vi "Analysis Test.vi"() -> ()   [LabVIEW 2017]
uses:
  Controller/Controller Data Cluster.ctl
  User Console/UI Data Cluster.ctl
  Controller/Timed Action.ctl
  Controller/Current Direction.ctl
  Controller/Communication/Controller Queue Message.ctl
panel:
  out "Current Direction":T1
  out "Controller Queue Message":T2=enum."Start and Move"
  in  "Controller Data Cluster 2":T3={"UI Data Cluster"={"Floor Selection"=[], "Elevator Call Up"=[], "Elevator Call Down"=[], "Door Buttons"={"Open"=FALSE, "Close"=FALSE}, "Emergency"=FALSE}, "Sensor Position"=1, "Module Closed?"={"Display Loop"=FALSE, "Sensor Loop "=FALSE}, "Time to Elapse"=0, "Request?"=FALSE, "Timed Action"=enum."Open Door", "Time Constants"={"Open Door"=5.0, "Close Door"=1.0, "Travel"=10.0, "Inactivity"=20.0}, "Inactivity"=FALSE, "Current Floor"=1, "Current Direction"=enum."Idle", "Travel?"=FALSE, "Program Exit"=[], "Emergency?"=FALSE}
  out "Error In 2":errorcluster
  in  "Error In":errorcluster
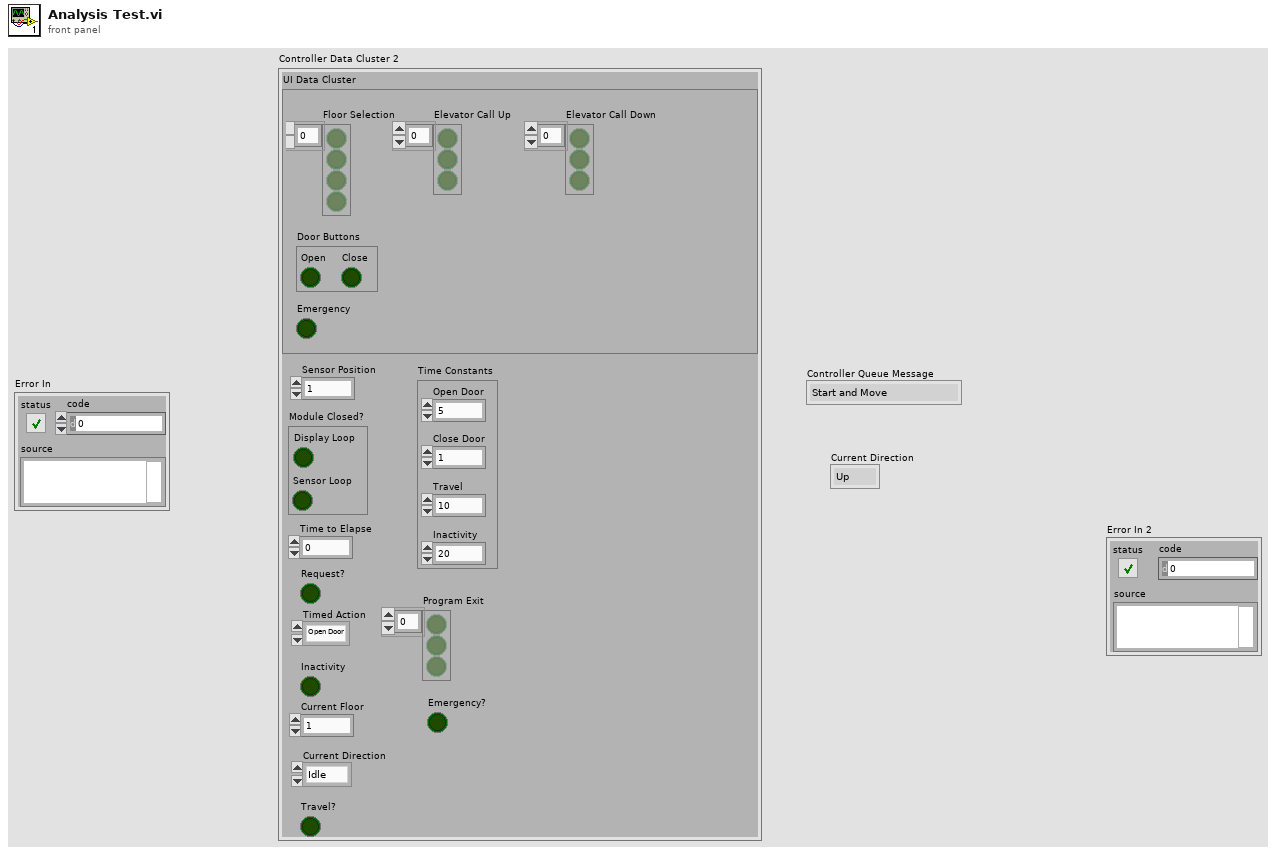
[diagram p1: front panel]
types:
  T1 = typedef "Current Direction.ctl" = enum16{"Up", "Down", "Idle"}
  T2 = typedef "Controller Queue Message.ctl" = enum16{"Initialize", "User Console Update", "Sensor Update", "Wait for First Request", "Start and Move", "Analysis", "Continue Travel", "Stop at Floor", "Open and Close Door Sequence", "Close Door", "No Request Remaining", "Check Time", "Emergency Call", "Terminate Process", "Start Exit", "Error Handling"}
  T3 = typedef "Controller Data Cluster.ctl" = cluster{"UI Data Cluster":T4, "Sensor Position":u32, "Module Closed?":cluster{"Display Loop":bool, "Sensor Loop ":bool}, "Time to Elapse":u32, "Request?":bool, "Timed Action":T5, "Time Constants":cluster{"Open Door":dbl, "Close Door":dbl, "Travel":dbl, "Inactivity":dbl}, "Inactivity":bool, "Current Floor":u32, "Current Direction":T1, "Travel?":bool, "Program Exit":bool[], "Emergency?":bool}
  T4 = typedef "UI Data Cluster.ctl" = cluster{"Floor Selection":bool[], "Elevator Call Up":bool[], "Elevator Call Down":bool[], "Door Buttons":cluster{"Open":bool, "Close":bool}, "Emergency":bool}
  T5 = typedef "Timed Action.ctl" = enum16{"Open Door", "Close Door", "Travel", "Inactivity"}
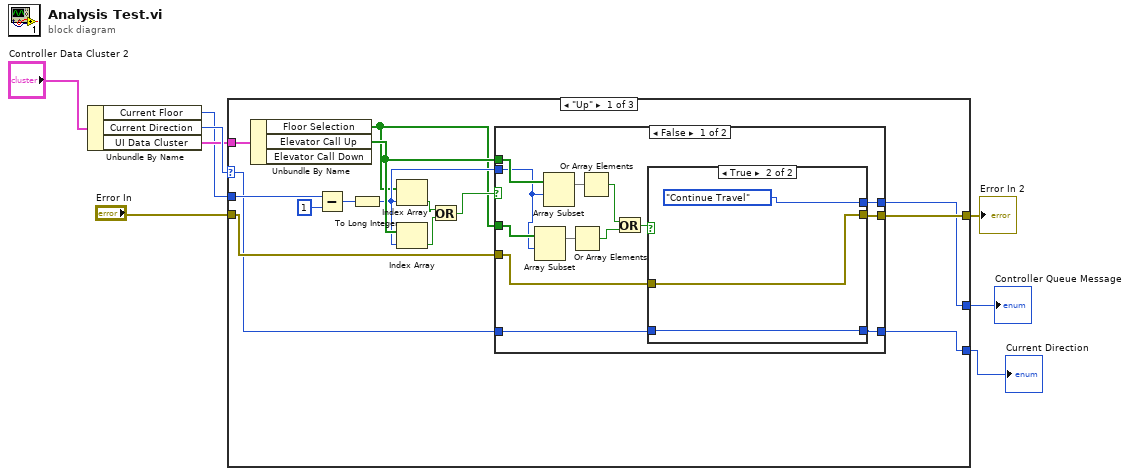
[diagram p0: block diagram]
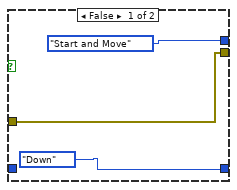
[diagram p2: hidden frame]
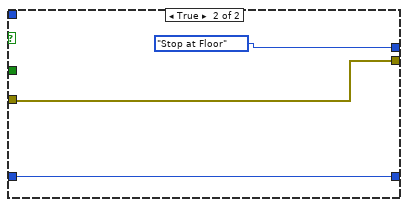
[diagram p3: hidden frame]
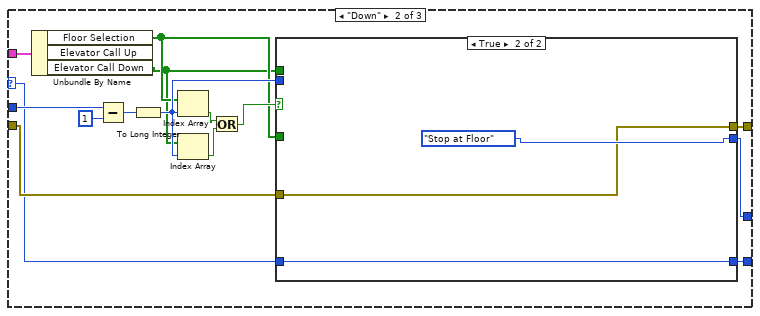
[diagram p4: hidden frame]
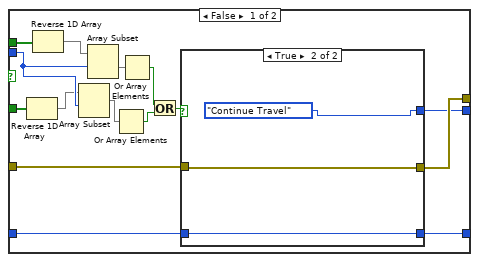
[diagram p5: hidden frame]
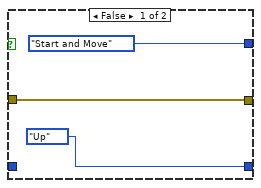
[diagram p6: hidden frame]
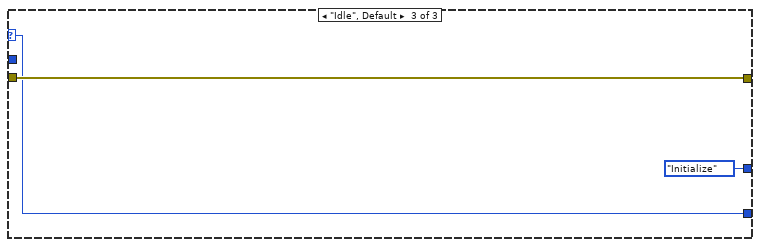
[diagram p7: hidden frame]
diagram:
  n1 = Unbundle By Name("Controller Data Cluster 2") -> ("Current Floor"=w6:u32, "Current Direction"=w8:T1, "UI Data Cluster"=w7:T4)
  n2 = case shown="\"Up\"" w8 {
    selector: w8 -> [w9 w46 w85]
    tunnel: "Error In" -> [w16 w53 w87]
    tunnel: [w15 w52 w87] -> w3
    tunnel: w7 -> [w22 w59 _]
    tunnel: w6 -> [w21 w58 _]
    tunnel: [w11 w48 Controller_Queue_Message."Initialize" ("Controller Queue Message")] -> w2
    tunnel: [w10 w47 w85] -> w1
    frame "Up" {
      n3 = Unbundle By Name(w22) -> ("Floor Selection"=w12:bool[], "Elevator Call Up"=w14:bool[])  [unwired: 1 out]
      n4 = Subtract(x=w21, y=u32 1) -> (x-y=w23:u32)
      n5 = To Long Integer(number=w23) -> (32bit integer=w13:i32)
      n6 = Index Array(array=w12, index=w13) -> (element=w19:bool)
      n7 = Index Array(array=w14, index=w13) -> (element=w18:bool)
      n8 = Or(x=w19, y=w18) -> (x .or. y?=w17:bool)
      n9 = case shown="False" w17 {
        tunnel: w16 -> [w28 w44]
        tunnel: [w27 w44] -> w15
        tunnel: w14 -> [w36 _]
        tunnel: w13 -> [w32 _]
        tunnel: w12 -> [w33 _]
        tunnel: [w26 Controller_Queue_Message."Stop at Floor" ("Controller Queue Message")] -> w11
        tunnel: [w25 w43] -> w10
        tunnel: w9 -> [w24 w43]
        frame False {
          n10 = Array Subset(array=w33, index=w32) -> (w34:bool[])  [unwired: 1 in]
          n11 = Array Subset(array=w36, index=w32) -> (w35:bool[])  [unwired: 1 in]
          n12 = Or Array Elements(Boolean array=w34) -> (logical OR=w30:bool)
          n13 = Or Array Elements(Boolean array=w35) -> (logical OR=w31:bool)
          n14 = Or(x=w31, y=w30) -> (x .or. y?=w29:bool)
          n15 = case shown="True" w29 {
            tunnel: w28 -> [w38 w40]
            tunnel: [w38 w40] -> w27
            tunnel: [Controller_Queue_Message."Start and Move" ("Controller Queue Message") Controller_Queue_Message."Continue Travel" ("Controller Queue Message")] -> w26
            tunnel: [Current_Direction."Down" ("Current Direction") w42] -> w25
            tunnel: w24 -> [_ w42]
            frame False {
            }
            frame True {
            }
          }
        }
        frame True {
        }
      }
    }
    frame "Down" {
      n16 = Unbundle By Name(w59) -> ("Floor Selection"=w50:bool[], "Elevator Call Down"=w49:bool[])  [unwired: 1 out]
      n17 = Subtract(x=w58, y=u32 1) -> (x-y=w60:u32)
      n18 = To Long Integer(number=w60) -> (32bit integer=w51:i32)
      n19 = Index Array(array=w50, index=w51) -> (element=w56:bool)
      n20 = Index Array(array=w49, index=w51) -> (element=w55:bool)
      n21 = Or(x=w56, y=w55) -> (x .or. y?=w54:bool)
      n22 = case shown="True" w54 {
        tunnel: w53 -> [w65 w82]
        tunnel: [w64 w82] -> w52
        tunnel: w49 -> [w69 _]
        tunnel: w51 -> [w73 _]
        tunnel: w50 -> [w67 _]
        tunnel: [w63 Controller_Queue_Message."Stop at Floor" ("Controller Queue Message")] -> w48
        tunnel: [w62 w84] -> w47
        tunnel: w46 -> [w61 w84]
        frame False {
          n23 = Reverse 1D Array(array=w67) -> (reversed array=w66:bool[])
          n24 = Reverse 1D Array(array=w69) -> (reversed array=w68:bool[])
          n25 = Array Subset(array=w66, index=w73) -> (w74:bool[])  [unwired: 1 in]
          n26 = Array Subset(array=w68, index=w73) -> (w75:bool[])  [unwired: 1 in]
          n27 = Or Array Elements(Boolean array=w74) -> (logical OR=w71:bool)
          n28 = Or Array Elements(Boolean array=w75) -> (logical OR=w72:bool)
          n29 = Or(x=w72, y=w71) -> (x .or. y?=w70:bool)
          n30 = case shown="True" w70 {
            tunnel: w65 -> [w78 w80]
            tunnel: [w78 w80] -> w64
            tunnel: [Controller_Queue_Message."Start and Move" ("Controller Queue Message") Controller_Queue_Message."Continue Travel" ("Controller Queue Message")] -> w63
            tunnel: [Current_Direction."Up" ("Current Direction") w79] -> w62
            tunnel: w61 -> [_ w79]
            frame False {
            }
            frame True {
            }
          }
        }
        frame True {
        }
      }
    }
    frame "Idle", Default {
    }
  }
  "Error In 2" <- w3
  "Controller Queue Message" <- w2
  "Current Direction" <- w1
